vi "K6514_DischargePreamp.vi"(8 "error in (no error)":errorcluster, 10 "discharge time (ms)":u32=250, 11 "VISA resource name in":refnum<visa-resource-name>) -> (0 "error out":errorcluster, 3 "VISA resource name out":refnum<visa-resource-name>)   [LabVIEW 2024]
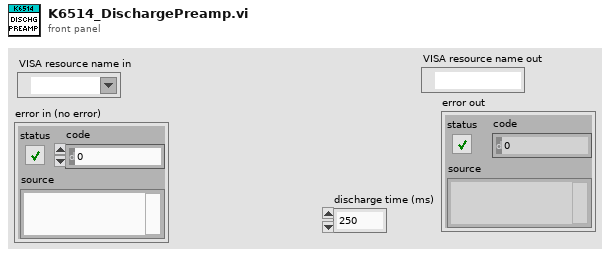
[diagram p1: front panel]
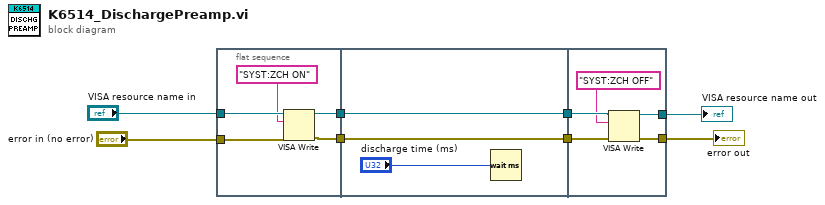
[diagram p0: block diagram]
diagram:
  n1 = flat-sequence {
    tunnel: "VISA resource name in" -> [w13]
    tunnel: [w12] -> w8
    tunnel: [w10] -> w6
    tunnel: "error in (no error)" -> [w9]
    tunnel: [w16] -> w7
    tunnel: w8 -> [w16]
    tunnel: w6 -> [w14]
    tunnel: [w14] -> w5
    tunnel: w7 -> [w21]
    tunnel: [w19] -> w2
    tunnel: [w18] -> w1
    tunnel: w5 -> [w17]
    frame #0 {
      n2 = VISA Write(VISA resource name=w13, write buffer="SYST:ZCH ON" ("String"), error in (no error)=w9) -> (VISA resource name out=w12:refnum<visa-resource-name>, error out=w10:errorcluster)  [unwired: 1 out]
    }
    frame #1 {
      n3 = Wait (ms)(milliseconds to wait="discharge time (ms)") -> ()  [unwired: 1 out]
    }
    frame #2 {
      n4 = VISA Write(VISA resource name=w21, write buffer="SYST:ZCH OFF", error in (no error)=w17) -> (VISA resource name out=w19:refnum<visa-resource-name>, error out=w18:errorcluster)  [unwired: 1 out]
    }
  }
  "VISA resource name out" <- w2
  "error out" <- w1
